vi "PH_SHS_Analysis_Calibrator.set initial state SM.vi"(0 "i ref in":refnum<vi>, 5 "error in (no error)":errorcluster) -> (14 "i ref out":refnum<vi>, 19 "error out":errorcluster)   [LabVIEW 2014, in "PH_SHS_Analysis_Calibrator.lvlib"]
doc: "This VI sets the initial state \"Stand by\"."
uses:
  PH_SHS_Analysis_Calibrator.lvlib
  CSCore/BaseSM/BaseSM.lvlib
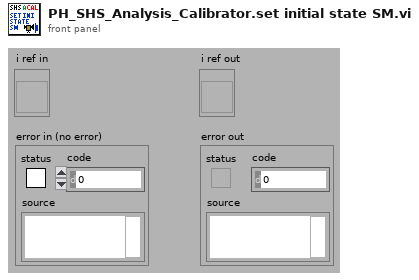
[diagram p1: front panel]
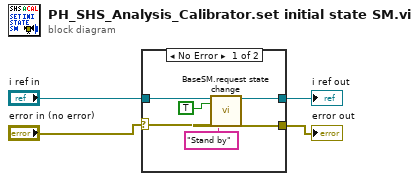
[diagram p0: block diagram]
diagram:
  n1 = case shown="No Error" "error in (no error)" {
    selector: "error in (no error)" -> [w5 w11]
    tunnel: "i ref in" -> [w10 w12]
    tunnel: [w9 w11] -> w4
    tunnel: [w6 w12] -> w1
    frame No Error {
      n2 = call "BaseSM.request state change.vi"("i ref in"=w10, "change"=TRUE, "error in (no error)"=w5, "requested state"="Stand by" ("next state")) -> ("i ref out"=w6:refnum<vi>, "error out"=w9:errorcluster)  [unwired: 12 in, 2 out]
    }
    frame Error {
    }
  }
  "error out" <- w4
  "i ref out" <- w1
